vi "TEMPLATE.vi"   [LabVIEW 2025, in "_Template.lvlib" / "Templates.lvlib" / "TEMPLATE jettl Actor.lvlib" / "TEMPLATE.lvlib"]
uses:
  TEMPLATE.lvlib
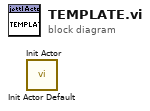
[diagram p0: block diagram]
diagram:
  n1 = call "Init Actor Default.vi"() -> ()  [unwired: 11 in, 1 out]
  n2 = call "Init Actor.vi"() -> ()  [unwired: 11 in, 1 out]
